vi "BASE-Main.vi"() -> ()   [LabVIEW 2017]
uses:
  <vilib>/Utility/error.llb/DialogType.ctl
panel:
  in  "MANUAL PRINT":bool
  in  "SETTING":bool
  in  "Torque IO Status":bool
  in  "Ass IO Status":bool
  in  "Recipe":bool
  out "error out":errorcluster
  in  "Logout":bool
  in  "Stop":bool
  in  "Create Login":bool
  in  "Reports":bool
  in  "Start":bool
  out "Time":string
  out "Date":string
  in  "Login":bool
  # "KAPSE SONS ROBOTICS\n& AUTOMATION"
  # "XBA ORVM"
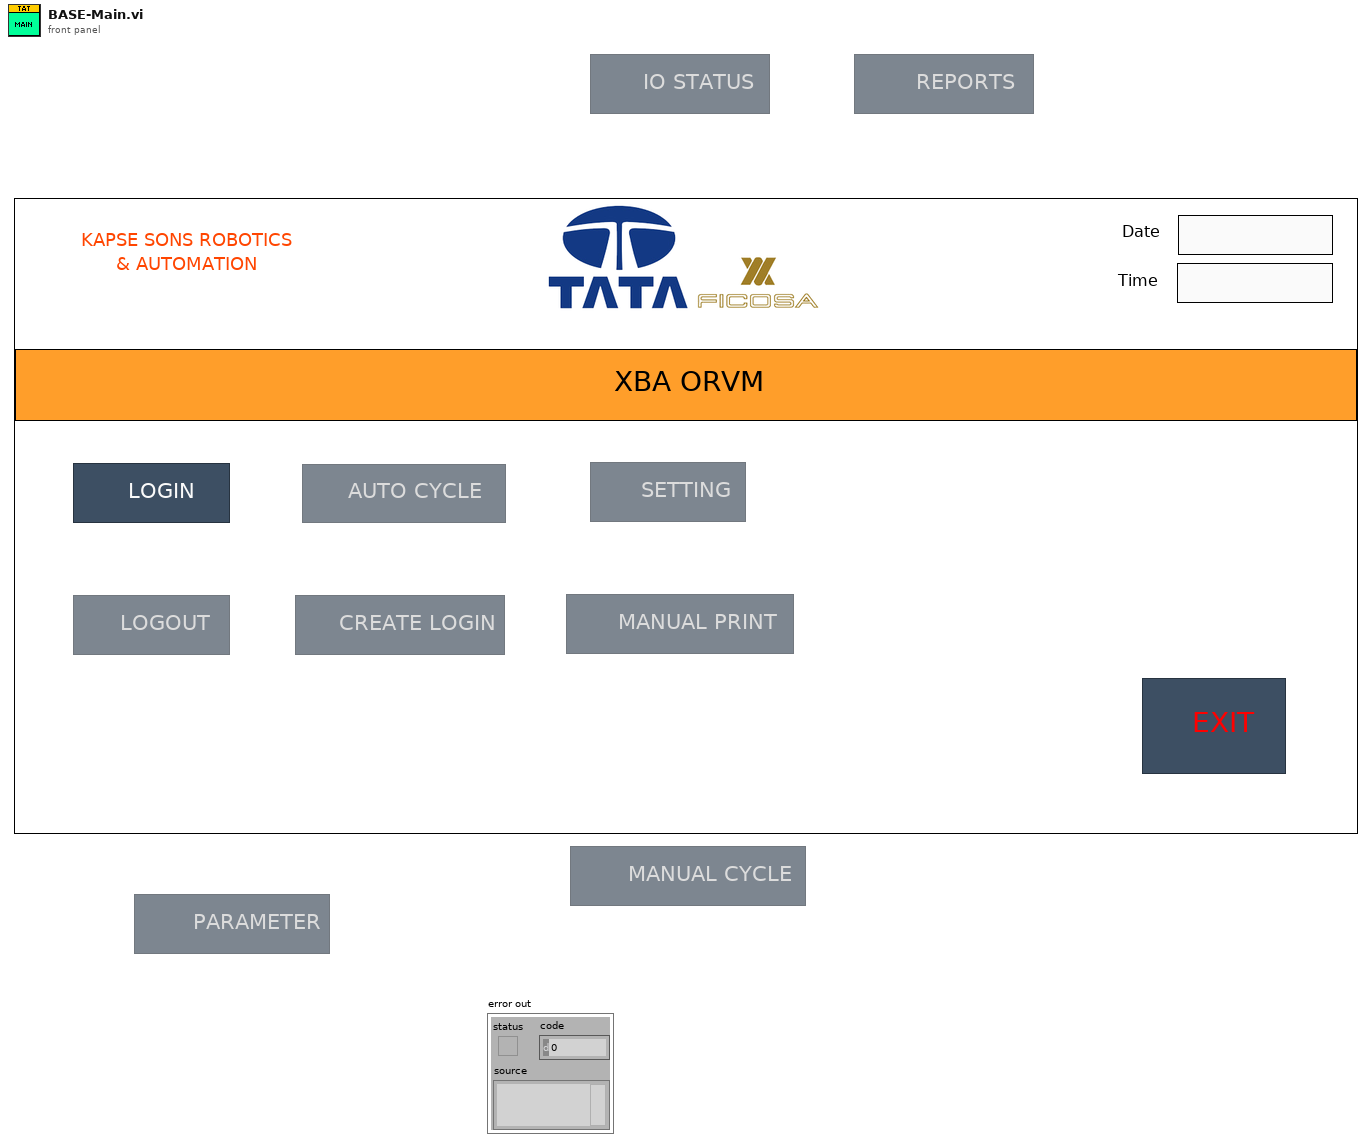
[diagram p1: front panel]
types:
  T1 = typedef "DialogType.ctl" = u16
  T2 = enum32{"Invalid", "Standard", "Closed", "Hidden", "Minimized", "Maximized"}
  T3 = enum8{"Enabled", "Disabled", "Disabled and Grayed Out"}
  T4 = enum32{"invalid app kind", "Development System", "Run Time System", "Student Edition", "Embedded LabVIEW", "Evaluation", "Custom"}
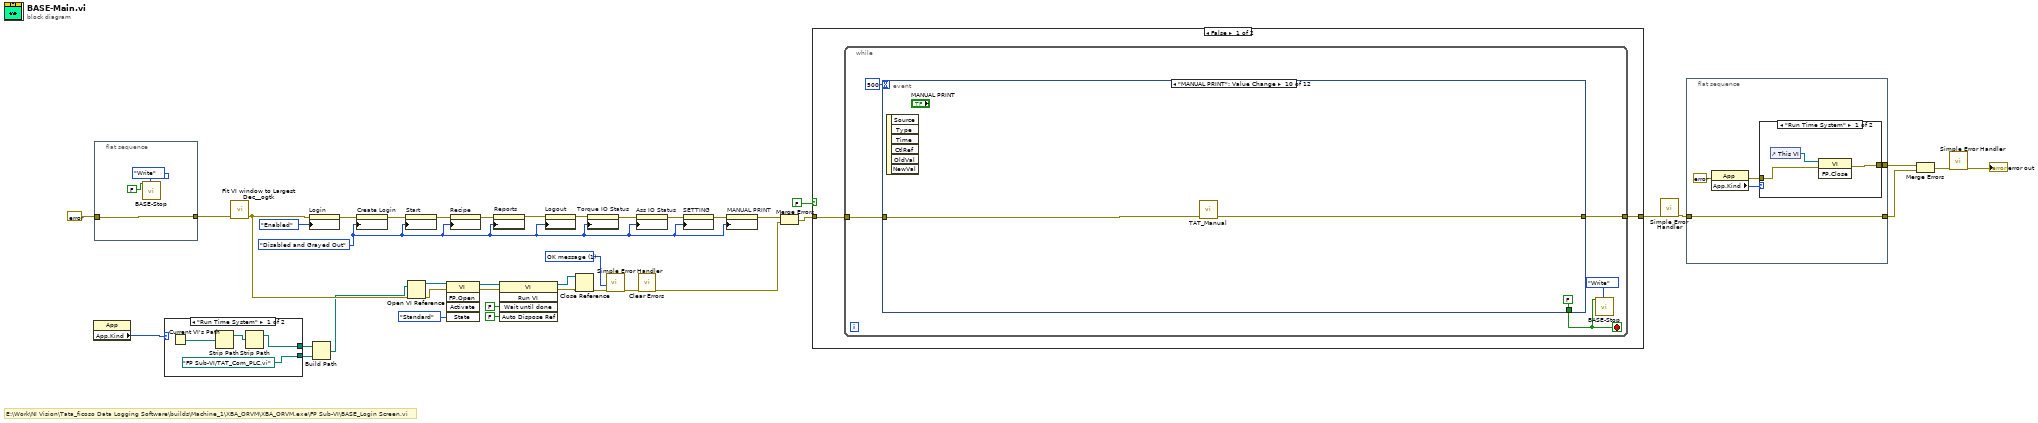
[diagram p0: block diagram]
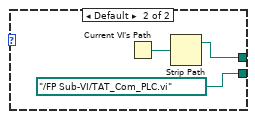
[diagram p2: hidden frame]
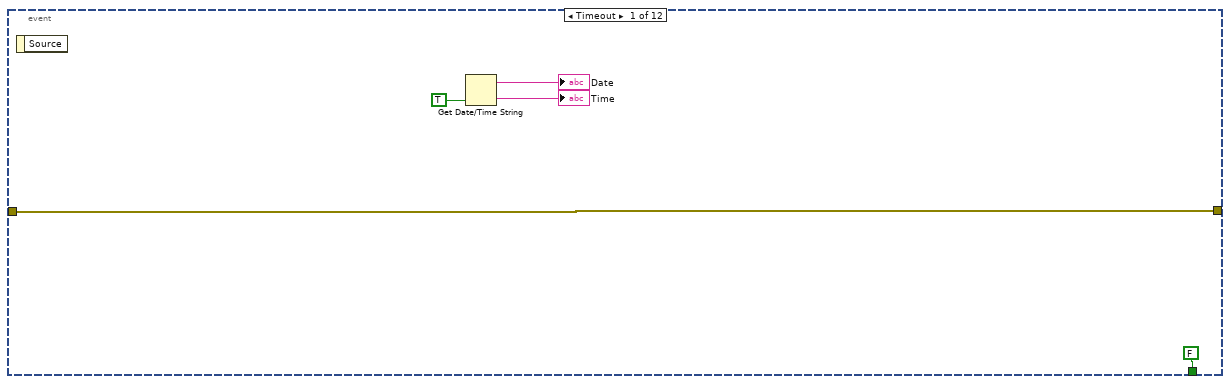
[diagram p4: hidden frame]
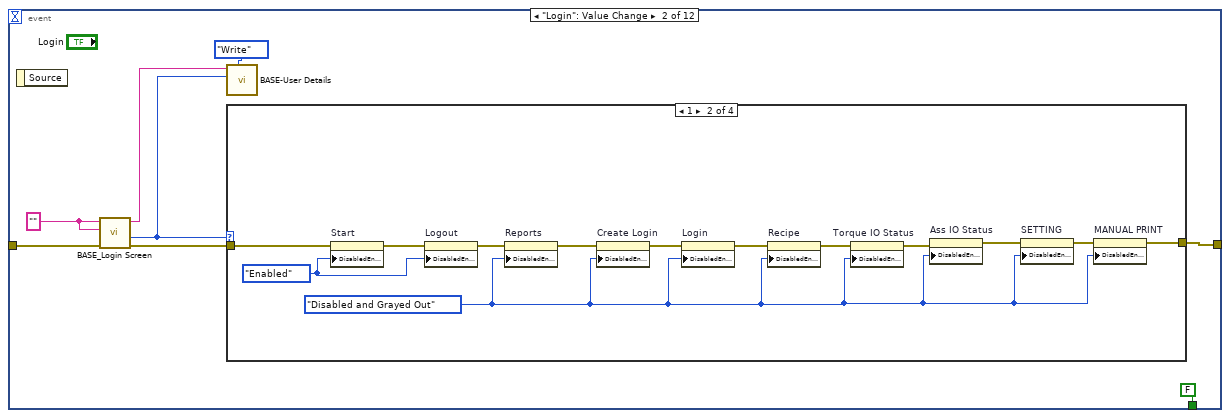
[diagram p5: hidden frame]
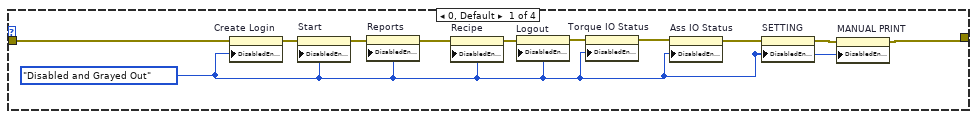
[diagram p6: hidden frame]
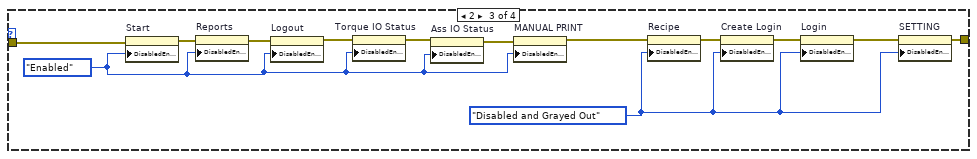
[diagram p7: hidden frame]
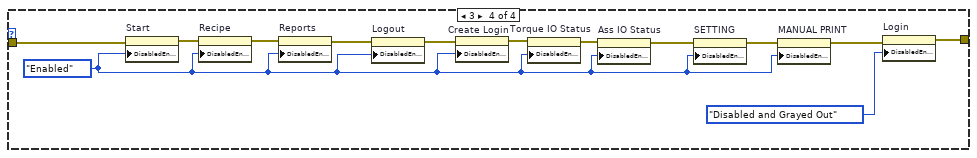
[diagram p8: hidden frame]
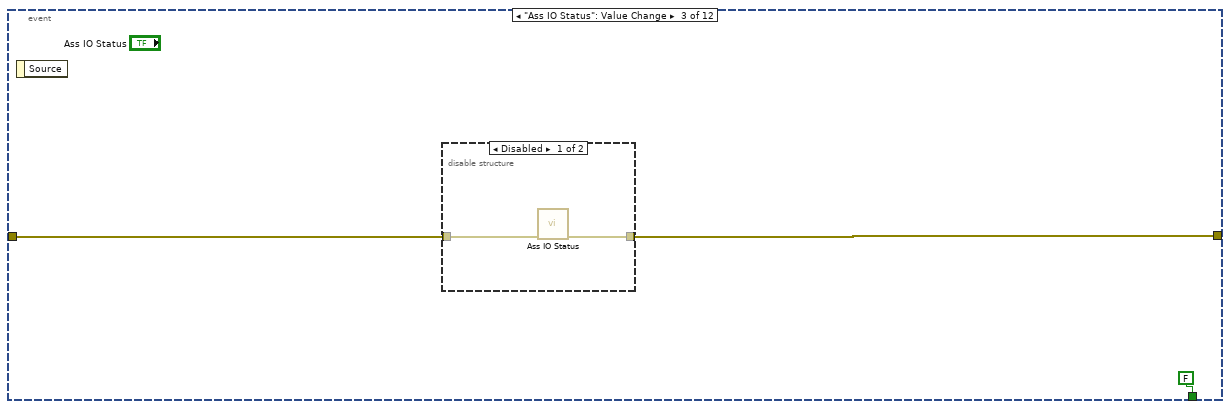
[diagram p9: hidden frame]
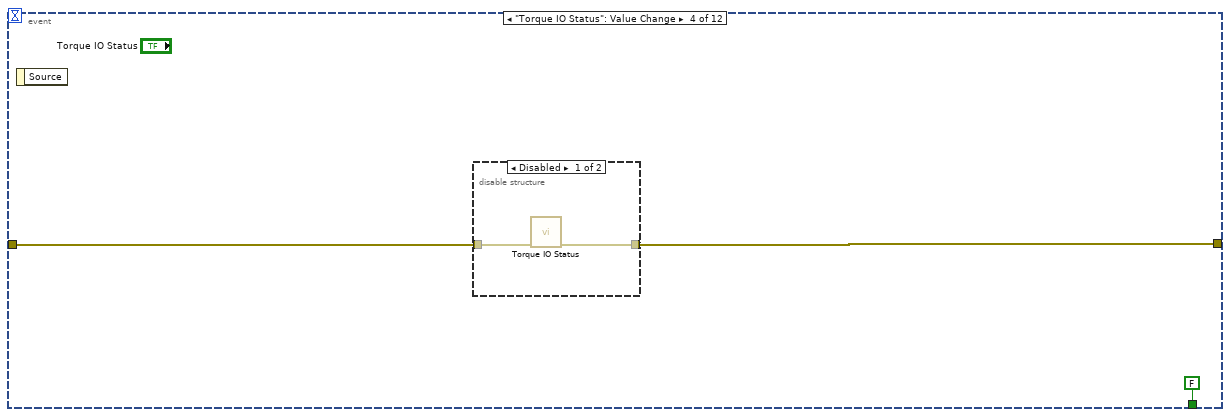
[diagram p11: hidden frame]
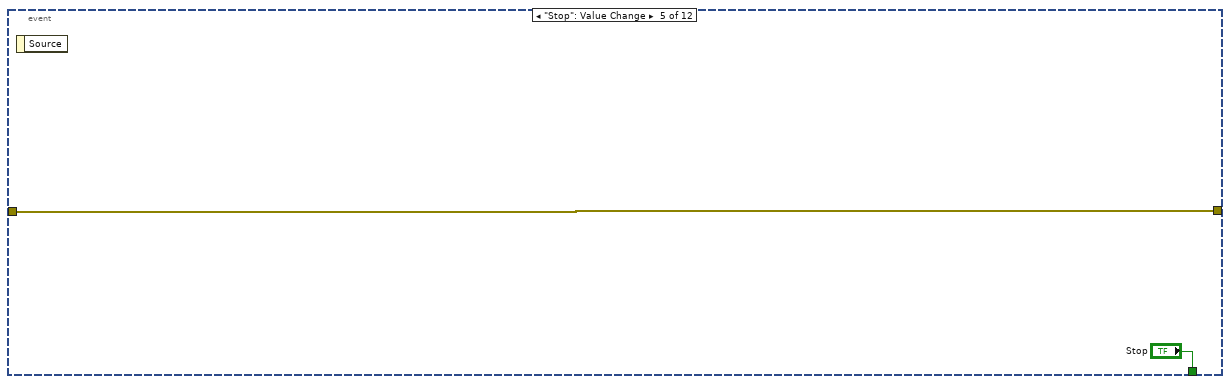
[diagram p13: hidden frame]
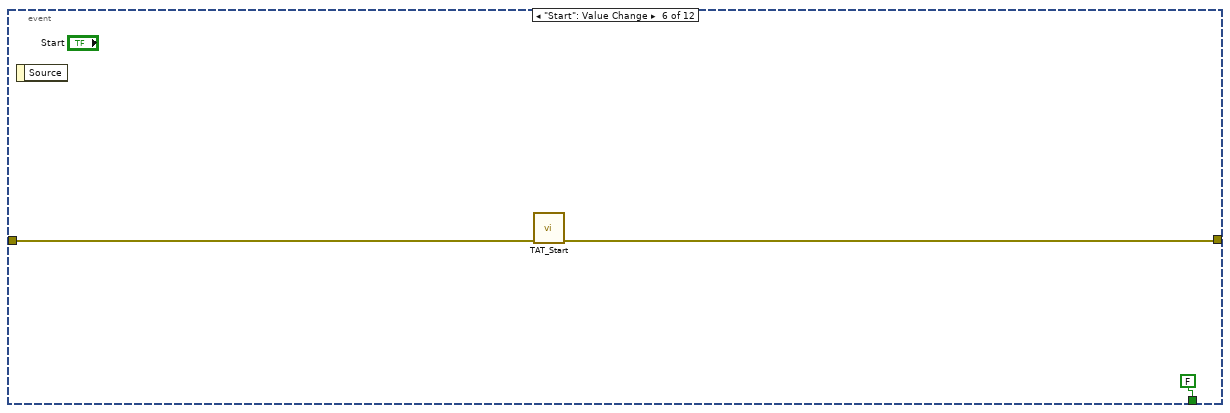
[diagram p14: hidden frame]
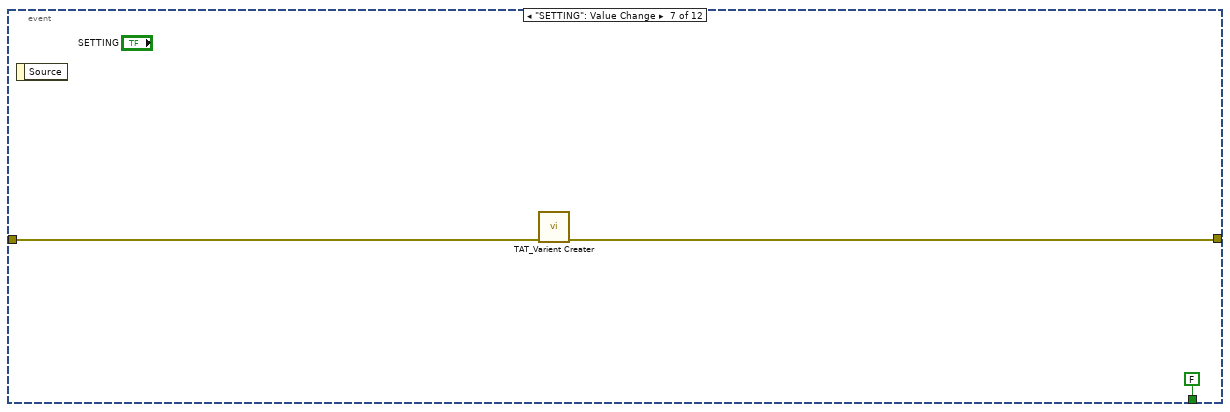
[diagram p15: hidden frame]
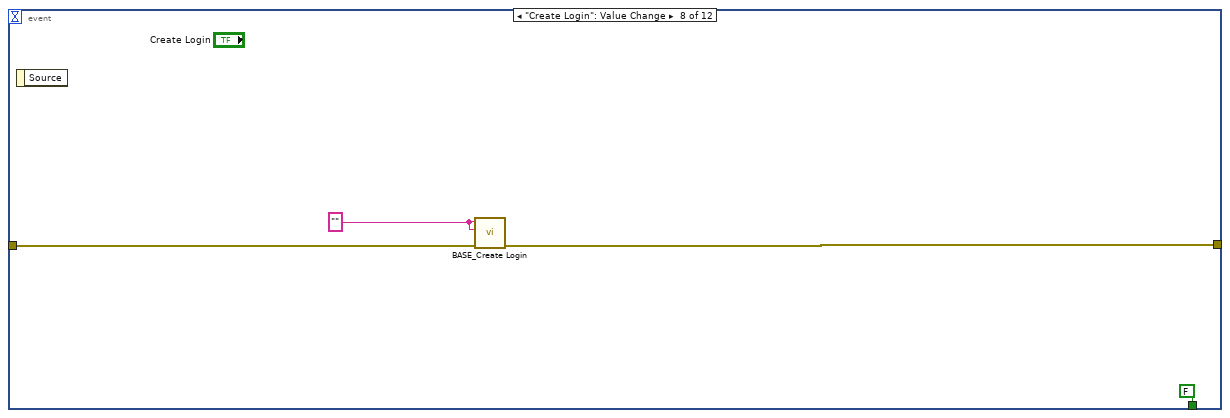
[diagram p16: hidden frame]
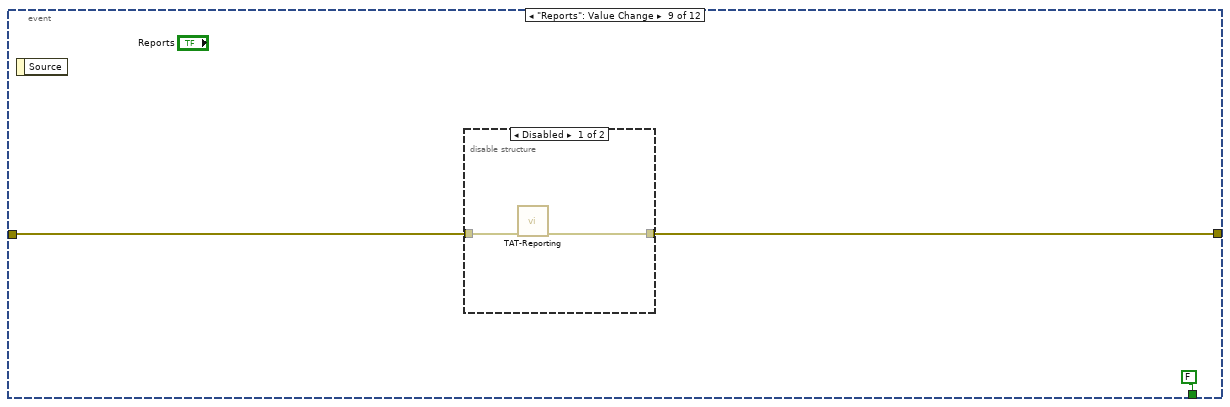
[diagram p17: hidden frame]
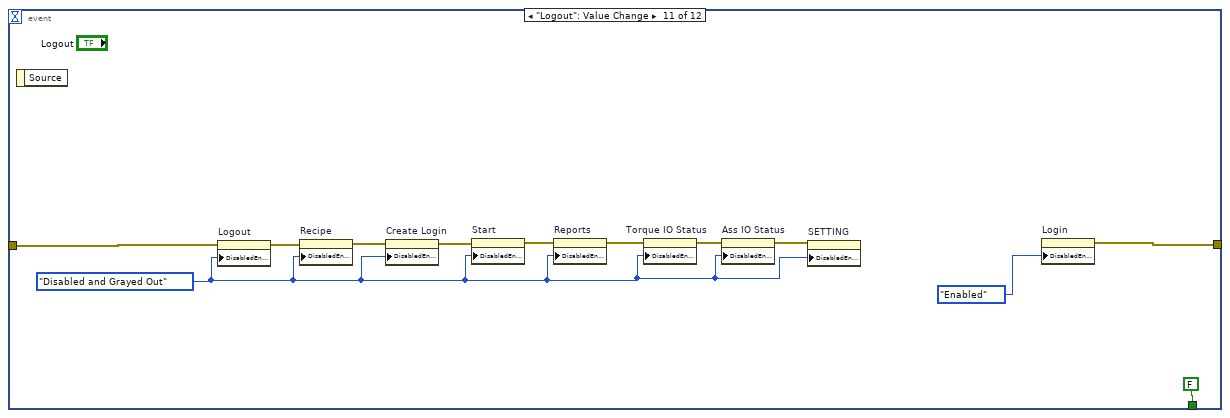
[diagram p19: hidden frame]
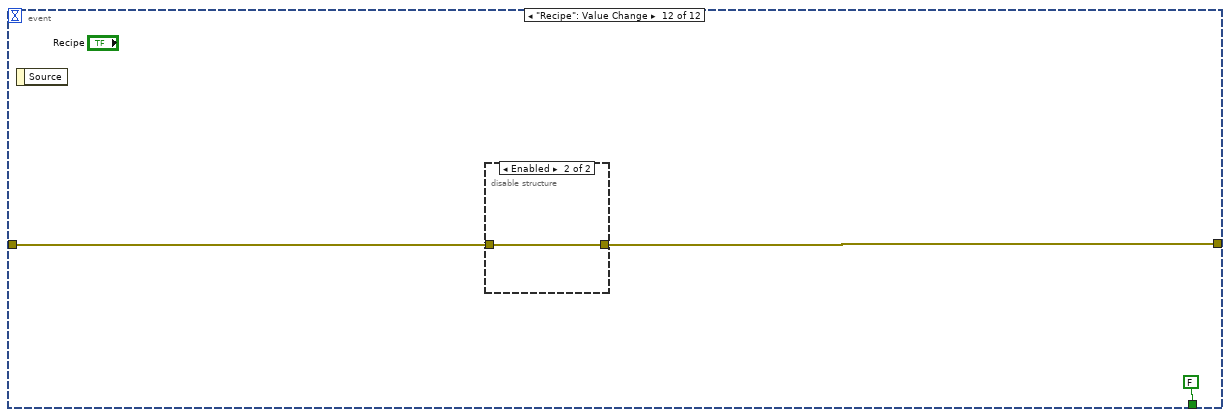
[diagram p20: hidden frame]
diagram:
  w11 = T1 1 items=["no dialog", "OK message", "continue or stop message", "OK message + warnings", "continue/stop + warnings"] ("type of dialog (OK msg:1)")
  w5 = T3."Disabled and Grayed Out" ("Disabled")
  # "E:\\Work\\NI Vision\\Tata_ficoso Data Logging Software\\builds\\Machine_1\\XBA_ORVM\\XBA_ORVM.exe\\FP Sub-VI\\BASE_Login Screen.vi"
  n1 = property class="App"() -> ("App.Kind"=w2:T4)  [unwired: 2 in, 2 out]
  n2 = flat-sequence {
    tunnel: [w43] -> w24
    tunnel: errorcluster {"status"=FALSE, "code"=0, "source"=""} ("error constant") -> [w43]
    frame #0 {
      n3 = call "BASE-Stop.vi"("Enum"=enum16{"Read", "Write"}."Write", "Stop"=FALSE) -> ()  [unwired: 9 in, 1 out]
    }
  }
  n4 = case shown="\"Run Time System\"" w2 {
    tunnel: [path "FP Sub-VI/TAT_Com_PLC.vi" ("path") path "../FP Sub-VI/TAT_Com_PLC.vi" ("path")] -> w3
    tunnel: [w44 w48] -> w4
    frame "Run Time System" {
      n5 = Current VI's Path() -> (path=w45:path)
      n6 = Strip Path(path=w45) -> (stripped path=w46:path)  [unwired: 1 out]
      n7 = Strip Path(path=w46) -> (stripped path=w44:path)  [unwired: 1 out]
    }
    frame Default {
      n8 = Current VI's Path() -> (path=w49:path)
      n9 = Strip Path(path=w49) -> (stripped path=w48:path)  [unwired: 1 out]
    }
  }
  n10 = call <userlib>:"Fit VI window to Largest Dec__ogtk.vi"("error in (no error)"=w24) -> ("error out"=w15:errorcluster)  [unwired: 5 in, 1 out]
  n11 = property on="Login" class="Bool"(error in=w15, "DisabledEnum"=T3."Enabled" ("Disabled")) -> (error out=w34:errorcluster)  [unwired: 1 in, 1 out]
  n12 = Build Path(base path=w4, name or relative path=w3) -> (appended path=w1:path)
  n13 = property on="Create Login" class="Bool"(error in=w34, "DisabledEnum"=w5) -> (error out=w39:errorcluster)  [unwired: 1 in, 1 out]
  n14 = property on="Start" class="Bool"(error in=w39, "DisabledEnum"=w5) -> (error out=w30:errorcluster)  [unwired: 1 in, 1 out]
  n15 = Open VI Reference(vi path=w1, error in (no error)=w15) -> (vi reference=w20:refnum<vi>, error out=w21:errorcluster)  [unwired: 4 in]
  n16 = invoke class="VI" method="FP.Open"(reference=w20, error in=w21, "State"=T2."Standard") -> (reference out=w23:refnum<vi>, error out=w22:errorcluster)  [unwired: 2 in, 3 out]
  n17 = property on="Recipe" class="Bool"(error in=w30, "DisabledEnum"=w5) -> (error out=w29:errorcluster)  [unwired: 1 in, 1 out]
  n18 = property on="Reports" class="Bool"(error in=w29, "DisabledEnum"=w5) -> (error out=w32:errorcluster)  [unwired: 1 in, 1 out]
  n19 = invoke class="VI" method="Run VI"(reference=w23, error in=w22, "Wait until done"=FALSE ("Wait Until Done"), "Auto Dispose Ref"=FALSE ("Auto Dispose Reference")) -> (reference out=w19:refnum<vi>, error out=w18:errorcluster)  [unwired: 1 in, 3 out]
  n20 = property on="Logout" class="Bool"(error in=w32, "DisabledEnum"=w5) -> (error out=w28:errorcluster)  [unwired: 1 in, 1 out]
  n21 = Close Reference(reference=w19, error in (no error)=w18) -> (error out=w12:errorcluster)
  n22 = property on="Torque IO Status" class="Bool"(error in=w28, "DisabledEnum"=w5) -> (error out=w27:errorcluster)  [unwired: 1 in, 1 out]
  n23 = call <vilib>:"Simple Error Handler.vi"("type of dialog (OK msg:1)"=w11, "error in (no error)"=w12) -> ("error out"=w10:errorcluster)  [unwired: 3 in, 4 out]
  n24 = property on="Ass IO Status" class="Bool"(error in=w27, "DisabledEnum"=w5) -> (error out=w26:errorcluster)  [unwired: 1 in, 1 out]
  n25 = call <vilib>:"Clear Errors.vi"("error in (no error)"=w10) -> ("error out"=w9:errorcluster)  [unwired: 5 in, 1 out]
  n26 = property on="SETTING" class="Bool"(error in=w26, "DisabledEnum"=w5) -> (error out=w7:errorcluster)  [unwired: 1 in, 1 out]
  n27 = property on="MANUAL PRINT" class="Bool"(error in=w7, "DisabledEnum"=w5) -> (error out=w6:errorcluster)  [unwired: 1 in, 1 out]
  n28 = Merge Errors(w6, w9) -> (w14:errorcluster)
  n29 = case shown="False" FALSE {
    tunnel: w14 -> [w52 w170]
    tunnel: [w51 w170] -> w40
    frame False {
      n30 = while {
        tunnel: w52 -> [w56]
        tunnel: [w55] -> w51
        stop <- w53 stop-if-true
        n31 = event shown="[9] \"MANUAL PRINT\": Value Change" {
          selector: _ -> [_ _ _ _ _ _ _ _ _ _ _ _]
          dyn-events: _ -> [_ _ _ _ _ _ _ _ _ _ _ _]
          timeout: 500 -> [_ _ _ _ _ _ _ _ _ _ _ _]
          tunnel: w56 -> [w60 w70 w123 w127 w132 w135 w138 w143 w146 w150 w160 w166]
          tunnel: [w60 w68 w122 w126 w132 w134 w137 w142 w145 w149 w161 w165] -> w55
          tunnel: [FALSE ("Stop") FALSE ("Stop") FALSE ("Stop") FALSE ("Stop") "Stop" FALSE ("Stop") FALSE ("Stop") FALSE ("Stop") FALSE ("Stop") FALSE ("Stop") FALSE ("Stop") FALSE ("Stop")] -> w53
          event Timeout {
            n32 = event-data() -> ()  [unwired: 1 in, 1 out]
            n33 = Get Date/Time String(want seconds? (F)=TRUE) -> (date string=→"Date":string, time string=→"Time":string)  [unwired: 2 in]
          }
          event "Login": Value Change {
            w65 = "" ("User Name")
            n34 = event-data() -> ()  [unwired: 1 in, 1 out]
            n35 = call "BASE_Login Screen.vi"("Error In"=w70, "Password"=w65, "User Name"=w65) -> ("error out"=w69:errorcluster, "Level"=w63:i32, "User Name Out"=w66:string)  [unwired: 5 in, 1 out]
            n36 = call "BASE-User Details.vi"("Enum"=enum16{"Read", "Write"}."Write", "Level In"=w63, "User Name In"=w66) -> ()  [unwired: 7 in, 2 out]
            n37 = case shown="1" w63 {
              tunnel: w69 -> [w79 w94 w107 w120]
              tunnel: [w72 w84 w98 w119] -> w68
              frame 0, Default {
                w71 = T3."Disabled and Grayed Out" ("Disabled")
                n38 = property on="Create Login" class="Bool"(error in=w79, "DisabledEnum"=w71) -> (error out=w81:errorcluster)  [unwired: 1 in, 1 out]
                n39 = property on="Start" class="Bool"(error in=w81, "DisabledEnum"=w71) -> (error out=w80:errorcluster)  [unwired: 1 in, 1 out]
                n40 = property on="Reports" class="Bool"(error in=w80, "DisabledEnum"=w71) -> (error out=w78:errorcluster)  [unwired: 1 in, 1 out]
                n41 = property on="Recipe" class="Bool"(error in=w78, "DisabledEnum"=w71) -> (error out=w77:errorcluster)  [unwired: 1 in, 1 out]
                n42 = property on="Logout" class="Bool"(error in=w77, "DisabledEnum"=w71) -> (error out=w76:errorcluster)  [unwired: 1 in, 1 out]
                n43 = property on="Torque IO Status" class="Bool"(error in=w76, "DisabledEnum"=w71) -> (error out=w75:errorcluster)  [unwired: 1 in, 1 out]
                n44 = property on="Ass IO Status" class="Bool"(error in=w75, "DisabledEnum"=w71) -> (error out=w74:errorcluster)  [unwired: 1 in, 1 out]
                n45 = property on="SETTING" class="Bool"(error in=w74, "DisabledEnum"=w71) -> (error out=w73:errorcluster)  [unwired: 1 in, 1 out]
                n46 = property on="MANUAL PRINT" class="Bool"(error in=w73, "DisabledEnum"=w71) -> (error out=w72:errorcluster)  [unwired: 1 in, 1 out]
              }
              frame 1 {
                w82 = T3."Disabled and Grayed Out" ("Disabled")
                w90 = T3."Enabled" ("Disabled")
                n47 = property on="Start" class="Bool"(error in=w94, "DisabledEnum"=w90) -> (error out=w89:errorcluster)  [unwired: 1 in, 1 out]
                n48 = property on="Logout" class="Bool"(error in=w89, "DisabledEnum"=w90) -> (error out=w92:errorcluster)  [unwired: 1 in, 1 out]
                n49 = property on="Reports" class="Bool"(error in=w92, "DisabledEnum"=w82) -> (error out=w93:errorcluster)  [unwired: 1 in, 1 out]
                n50 = property on="Create Login" class="Bool"(error in=w93, "DisabledEnum"=w82) -> (error out=w91:errorcluster)  [unwired: 1 in, 1 out]
                n51 = property on="Login" class="Bool"(error in=w91, "DisabledEnum"=w82) -> (error out=w88:errorcluster)  [unwired: 1 in, 1 out]
                n52 = property on="Recipe" class="Bool"(error in=w88, "DisabledEnum"=w82) -> (error out=w86:errorcluster)  [unwired: 1 in, 1 out]
                n53 = property on="Torque IO Status" class="Bool"(error in=w86, "DisabledEnum"=w82) -> (error out=w87:errorcluster)  [unwired: 1 in, 1 out]
                n54 = property on="Ass IO Status" class="Bool"(error in=w87, "DisabledEnum"=w82) -> (error out=w85:errorcluster)  [unwired: 1 in, 1 out]
                n55 = property on="SETTING" class="Bool"(error in=w85, "DisabledEnum"=w82) -> (error out=w83:errorcluster)  [unwired: 1 in, 1 out]
                n56 = property on="MANUAL PRINT" class="Bool"(error in=w83, "DisabledEnum"=w82) -> (error out=w84:errorcluster)  [unwired: 1 in, 1 out]
              }
              frame 2 {
                w99 = T3."Disabled and Grayed Out" ("Disabled")
                w95 = T3."Enabled" ("Disabled")
                n57 = property on="Start" class="Bool"(error in=w107, "DisabledEnum"=w95) -> (error out=w104:errorcluster)  [unwired: 1 in, 1 out]
                n58 = property on="Reports" class="Bool"(error in=w104, "DisabledEnum"=w95) -> (error out=w106:errorcluster)  [unwired: 1 in, 1 out]
                n59 = property on="Logout" class="Bool"(error in=w106, "DisabledEnum"=w95) -> (error out=w101:errorcluster)  [unwired: 1 in, 1 out]
                n60 = property on="Torque IO Status" class="Bool"(error in=w101, "DisabledEnum"=w95) -> (error out=w102:errorcluster)  [unwired: 1 in, 1 out]
                n61 = property on="Ass IO Status" class="Bool"(error in=w102, "DisabledEnum"=w95) -> (error out=w97:errorcluster)  [unwired: 1 in, 1 out]
                n62 = property on="MANUAL PRINT" class="Bool"(error in=w97, "DisabledEnum"=w95) -> (error out=w96:errorcluster)  [unwired: 1 in, 1 out]
                n63 = property on="Recipe" class="Bool"(error in=w96, "DisabledEnum"=w99) -> (error out=w103:errorcluster)  [unwired: 1 in, 1 out]
                n64 = property on="Create Login" class="Bool"(error in=w103, "DisabledEnum"=w99) -> (error out=w105:errorcluster)  [unwired: 1 in, 1 out]
                n65 = property on="Login" class="Bool"(error in=w105, "DisabledEnum"=w99) -> (error out=w100:errorcluster)  [unwired: 1 in, 1 out]
                n66 = property on="SETTING" class="Bool"(error in=w100, "DisabledEnum"=w99) -> (error out=w98:errorcluster)  [unwired: 1 in, 1 out]
              }
              frame 3 {
                w108 = T3."Enabled" ("Disabled")
                n67 = property on="Start" class="Bool"(error in=w120, "DisabledEnum"=w108) -> (error out=w115:errorcluster)  [unwired: 1 in, 1 out]
                n68 = property on="Recipe" class="Bool"(error in=w115, "DisabledEnum"=w108) -> (error out=w114:errorcluster)  [unwired: 1 in, 1 out]
                n69 = property on="Reports" class="Bool"(error in=w114, "DisabledEnum"=w108) -> (error out=w117:errorcluster)  [unwired: 1 in, 1 out]
                n70 = property on="Logout" class="Bool"(error in=w117, "DisabledEnum"=w108) -> (error out=w116:errorcluster)  [unwired: 1 in, 1 out]
                n71 = property on="Create Login" class="Bool"(error in=w116, "DisabledEnum"=w108) -> (error out=w113:errorcluster)  [unwired: 1 in, 1 out]
                n72 = property on="Torque IO Status" class="Bool"(error in=w113, "DisabledEnum"=w108) -> (error out=w112:errorcluster)  [unwired: 1 in, 1 out]
                n73 = property on="Ass IO Status" class="Bool"(error in=w112, "DisabledEnum"=w108) -> (error out=w111:errorcluster)  [unwired: 1 in, 1 out]
                n74 = property on="SETTING" class="Bool"(error in=w111, "DisabledEnum"=w108) -> (error out=w110:errorcluster)  [unwired: 1 in, 1 out]
                n75 = property on="MANUAL PRINT" class="Bool"(error in=w110, "DisabledEnum"=w108) -> (error out=w109:errorcluster)  [unwired: 1 in, 1 out]
                n76 = property on="Login" class="Bool"(error in=w109, "DisabledEnum"=T3."Disabled and Grayed Out" ("Disabled")) -> (error out=w119:errorcluster)  [unwired: 1 in, 1 out]
              }
            }
          }
          event "Ass IO Status": Value Change {
            n77 = event-data() -> ()  [unwired: 1 in, 1 out]
            n78 = disable-structure shown="Disabled" {
              disable-tunnel: w123 -> [w125 _]
              disable-tunnel: [w124 _] -> w122
              frame Disabled {
                n79 = call "Ass IO Status.vi"("error in (no error)"=w125) -> ("error out"=w124:errorcluster)  [unwired: 10 in]
              }
              frame Enabled {
              }
            }
          }
          event "Torque IO Status": Value Change {
            n80 = event-data() -> ()  [unwired: 1 in, 1 out]
            n81 = disable-structure shown="Disabled" {
              disable-tunnel: w127 -> [w130 w131]
              disable-tunnel: [w129 w131] -> w126
              frame Disabled {
                n82 = call "Torque IO Status.vi"("error in (no error)"=w130) -> ("error out"=w129:errorcluster)  [unwired: 10 in]
              }
              frame Enabled {
              }
            }
          }
          event "Stop": Value Change {
            n83 = event-data() -> ()  [unwired: 1 in, 1 out]
          }
          event "Start": Value Change {
            n84 = event-data() -> ()  [unwired: 1 in, 1 out]
            n85 = call "TAT_Start.vi"("error In"=w135) -> ("error out"=w134:errorcluster)  [unwired: 10 in]
          }
          event "SETTING": Value Change {
            n86 = event-data() -> ()  [unwired: 1 in, 1 out]
            n87 = call "TAT_Varient Creater.vi"("error in (no error)"=w138) -> ("error out"=w137:errorcluster)  [unwired: 10 in]
          }
          event "Create Login": Value Change {
            w141 = "" ("User Name")
            n88 = event-data() -> ()  [unwired: 1 in, 1 out]
            n89 = call "BASE_Create Login.vi"("Error In"=w143, "Password"=w141, "User Name"=w141) -> ("error out"=w142:errorcluster)  [unwired: 6 in]
          }
          event "Reports": Value Change {
            n90 = event-data() -> ()  [unwired: 1 in, 1 out]
            n91 = disable-structure shown="Disabled" {
              disable-tunnel: w146 -> [w148 _]
              disable-tunnel: [w147 _] -> w145
              frame Disabled {
                n92 = call "TAT-Reporting.vi"("error in (no error)"=w148) -> ("error out"=w147:errorcluster)  [unwired: 10 in]
              }
              frame Enabled {
              }
            }
          }
          event "MANUAL PRINT": Value Change {
            n93 = event-data() -> ()  [unwired: 1 in, 6 out]
            n94 = call "TAT_Manual.vi"("error In"=w150) -> ("error out"=w149:errorcluster)  [unwired: 10 in]
          }
          event "Logout": Value Change {
            w152 = T3."Disabled and Grayed Out" ("Disabled")
            n95 = event-data() -> ()  [unwired: 1 in, 1 out]
            n96 = property on="Logout" class="Bool"(error in=w160, "DisabledEnum"=w152) -> (error out=w158:errorcluster)  [unwired: 1 in, 1 out]
            n97 = property on="Recipe" class="Bool"(error in=w158, "DisabledEnum"=w152) -> (error out=w157:errorcluster)  [unwired: 1 in, 1 out]
            n98 = property on="Create Login" class="Bool"(error in=w157, "DisabledEnum"=w152) -> (error out=w163:errorcluster)  [unwired: 1 in, 1 out]
            n99 = property on="Start" class="Bool"(error in=w163, "DisabledEnum"=w152) -> (error out=w162:errorcluster)  [unwired: 1 in, 1 out]
            n100 = property on="Reports" class="Bool"(error in=w162, "DisabledEnum"=w152) -> (error out=w155:errorcluster)  [unwired: 1 in, 1 out]
            n101 = property on="Torque IO Status" class="Bool"(error in=w155, "DisabledEnum"=w152) -> (error out=w156:errorcluster)  [unwired: 1 in, 1 out]
            n102 = property on="Ass IO Status" class="Bool"(error in=w156, "DisabledEnum"=w152) -> (error out=w153:errorcluster)  [unwired: 1 in, 1 out]
            n103 = property on="SETTING" class="Bool"(error in=w153, "DisabledEnum"=w152) -> ()  [unwired: 1 in, 2 out]
            n104 = property on="Login" class="Bool"("DisabledEnum"=T3."Enabled" ("Disabled")) -> (error out=w161:errorcluster)  [unwired: 2 in, 1 out]
          }
          event "Recipe": Value Change {
            n105 = event-data() -> ()  [unwired: 1 in, 1 out]
            n106 = disable-structure shown="Enabled" {
              disable-tunnel: w166 -> [w168 w169]
              disable-tunnel: [w167 w169] -> w165
              frame Disabled {
                n107 = call "TAT-Create Reciepe.vi"("Error In"=w168) -> ("error out"=w167:errorcluster)  [unwired: 10 in]
              }
              frame Enabled {
              }
            }
          }
        }
        n108 = call "BASE-Stop.vi"("Enum"=enum16{"Read", "Write"}."Write", "Stop"=w53) -> ()  [unwired: 9 in, 1 out]
      }
    }
    frame True {
    }
  }
  n109 = call <vilib>:"Simple Error Handler.vi"("error in (no error)"=w40) -> ("error out"=w35:errorcluster)  [unwired: 4 in, 4 out]
  n110 = flat-sequence {
    tunnel: [w172] -> w38
    tunnel: [w171] -> w36
    tunnel: w35 -> [w171]
    frame #0 {
      n111 = property class="App"(error in=errorcluster {"status"=FALSE, "code"=0, "source"=""} ("error in (no error)")) -> (error out=w174:errorcluster, "App.Kind"=w175:T4)  [unwired: 1 in, 1 out]
      n112 = case shown="\"Run Time System\"" w175 {
        tunnel: w174 -> [w177 w179]
        tunnel: [w176 w179] -> w172
        frame "Run Time System" {
          n113 = control-ref of="This VI"() -> (w178:refnum<vi>)
          n114 = invoke class="VI" method="FP.Close"(reference=w178, error in=w177) -> (error out=w176:errorcluster)  [unwired: 1 in, 2 out]
        }
        frame "Development System", Default {
        }
      }
    }
  }
  n115 = Merge Errors(w38, w36) -> (w37:errorcluster)
  n116 = call <vilib>:"Simple Error Handler.vi"("error in (no error)"=w37) -> ("error out"=→"error out":errorcluster)  [unwired: 4 in, 4 out]
